vi "Teststand Status FGV.vi"(8 "error in":errorcluster, 10 "Teststand Status":T1, 11 "Option":enum16{"Set", "Get"}(ring)) -> (0 "error out":errorcluster, 2 "Teststand Status Out":T1)   [LabVIEW 2023, in "HardwareAbstractionLayer_LVOOP.lvlib" / "Teststand.lvclass"]
doc: "This vi used to set and get teststand function global variables."
uses:
  Teststand.lvclass
  Control/Teststand Status Control.ctl
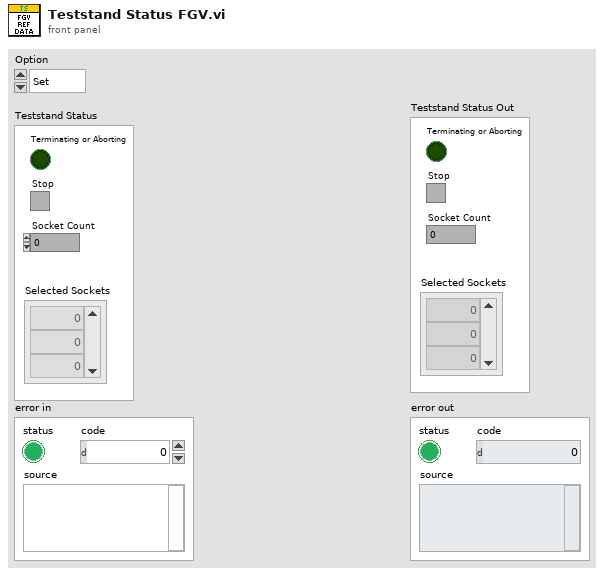
[diagram p1: front panel]
types:
  T1 = typedef "HardwareAbstractionLayer_LVOOP.lvlib/Teststand.lvclass/Teststand Status Control.ctl" = cluster{"Terminating or Aborting":bool, "Stop":bool, "Socket Count":i16, "Selected Sockets":i16[]}
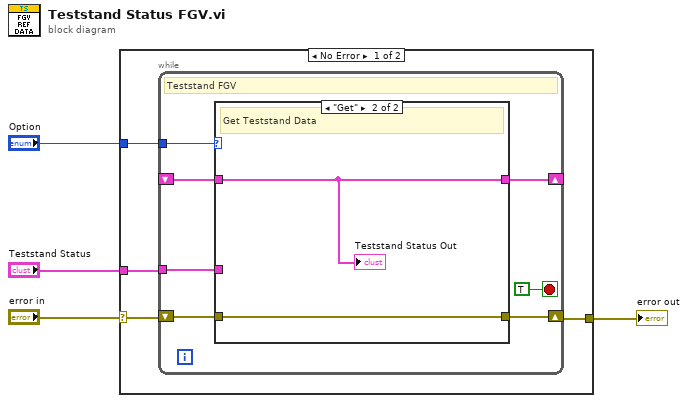
[diagram p0: block diagram]
diagram:
  n1 = case shown="No Error" "error in" {
    selector: "error in" -> [w7 w20]
    tunnel: "Option" -> [w8 _]
    tunnel: [w6 w20] -> w2
    tunnel: "Teststand Status" -> [w5 _]
    frame No Error {
      n2 = while {
        tunnel: w8 -> [w15]
        shift-right: [w12] -> w6
        shift-left: w7 -> [w13]
        tunnel: w5 -> [w11]
        shift-right: [w10] -> _
        shift-left: _ -> [w9]
        stop <- TRUE stop-if-true
        # "Teststand FGV"
        n3 = case shown="\"Get\"" w15 {
          tunnel: w13 -> [w17 w18]
          tunnel: [w17 w18] -> w12
          tunnel: w11 -> [w16 _]
          tunnel: [w16 w19] -> w10
          tunnel: w9 -> [_ w19]
          frame "Set", Default {
            # "Set Teststand Data"
          }
          frame "Get" {
            # "Get Teststand Data"
            "Teststand Status Out" <- w19
          }
        }
      }
    }
    frame Error {
    }
  }
  "error out" <- w2
